vi "Teleop.vi"(8 "error in (no error)":errorcluster, 11 "XboxController-V in":refnum<class "XboxController-V.lvclass">) -> (0 "error out":errorcluster, 3 "XboxController-V out":refnum<class "XboxController-V.lvclass">)   [LabVIEW 2013, in "XboxController-V.lvclass"]
uses:
  XboxController-V.lvclass
  XboxController-V.lvclass/XboxController-V.ctl
  Logical Systems/XBoxController/XBoxController.lvclass
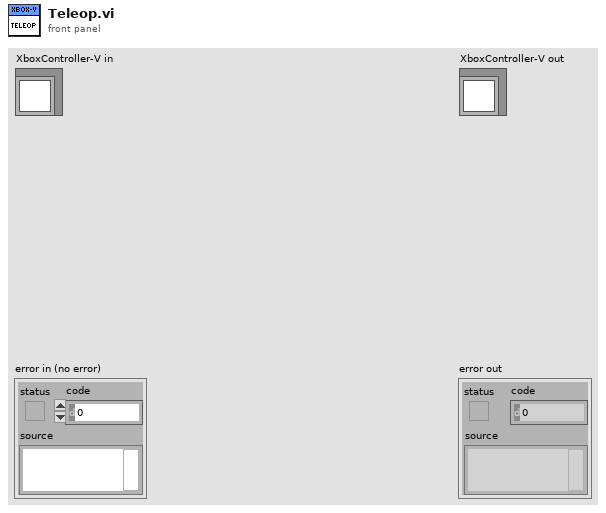
[diagram p1: front panel]
types:
  T1 = cluster{"Left Bumper":bool, "Right Bumper":bool, "Left Joystick Forward":dbl, "Left Joystick Right":dbl, "Right Joystick Forward":dbl, "Right Joystick Right":dbl}
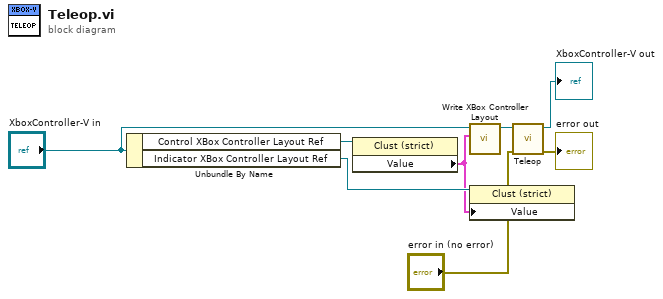
[diagram p0: block diagram]
diagram:
  n1 = Unbundle By Name("XboxController-V in") -> ("Control XBox Controller Layout Ref"=w6:refnum<vi>, "Indicator XBox Controller Layout Ref"=w3:refnum<vi>)
  n2 = property class="Clust (strict)"(reference=w6) -> ("Value"=w2:T1)  [unwired: 1 in, 2 out]
  n3 = call-dynamic "Write XBox Controller Layout.vi"("XBox Controller Layout"=w2, "XBoxController in"="XboxController-V in") -> ("XBoxController out"=w4:refnum<class "XboxController-V.lvclass">)  [unwired: 8 in, 1 out]
  n4 = property class="Clust (strict)"(reference=w3, "Value"=w2) -> ()  [unwired: 1 in, 2 out]
  n5 = call-parent "Teleop.vi"("error in (no error)"="error in (no error)", "XBoxController in"=w4) -> ("error out"=→"error out":errorcluster, "XBoxController out"=→"XboxController-V out":refnum<class "XboxController-V.lvclass">)  [unwired: 8 in]
